vi "Aquire AI Data.vi"() -> ()   [LabVIEW 2017]
panel:
  out "Table":string[](array[string])
  out "Chart":dbl(graph)
  # "采集时间"
  # "采集棒位二进制值"
  # "查表输出值"
  # "棒位理论值"
  # "光栅尺位置"
  # "光栅尺速度"
  # "移动方向"
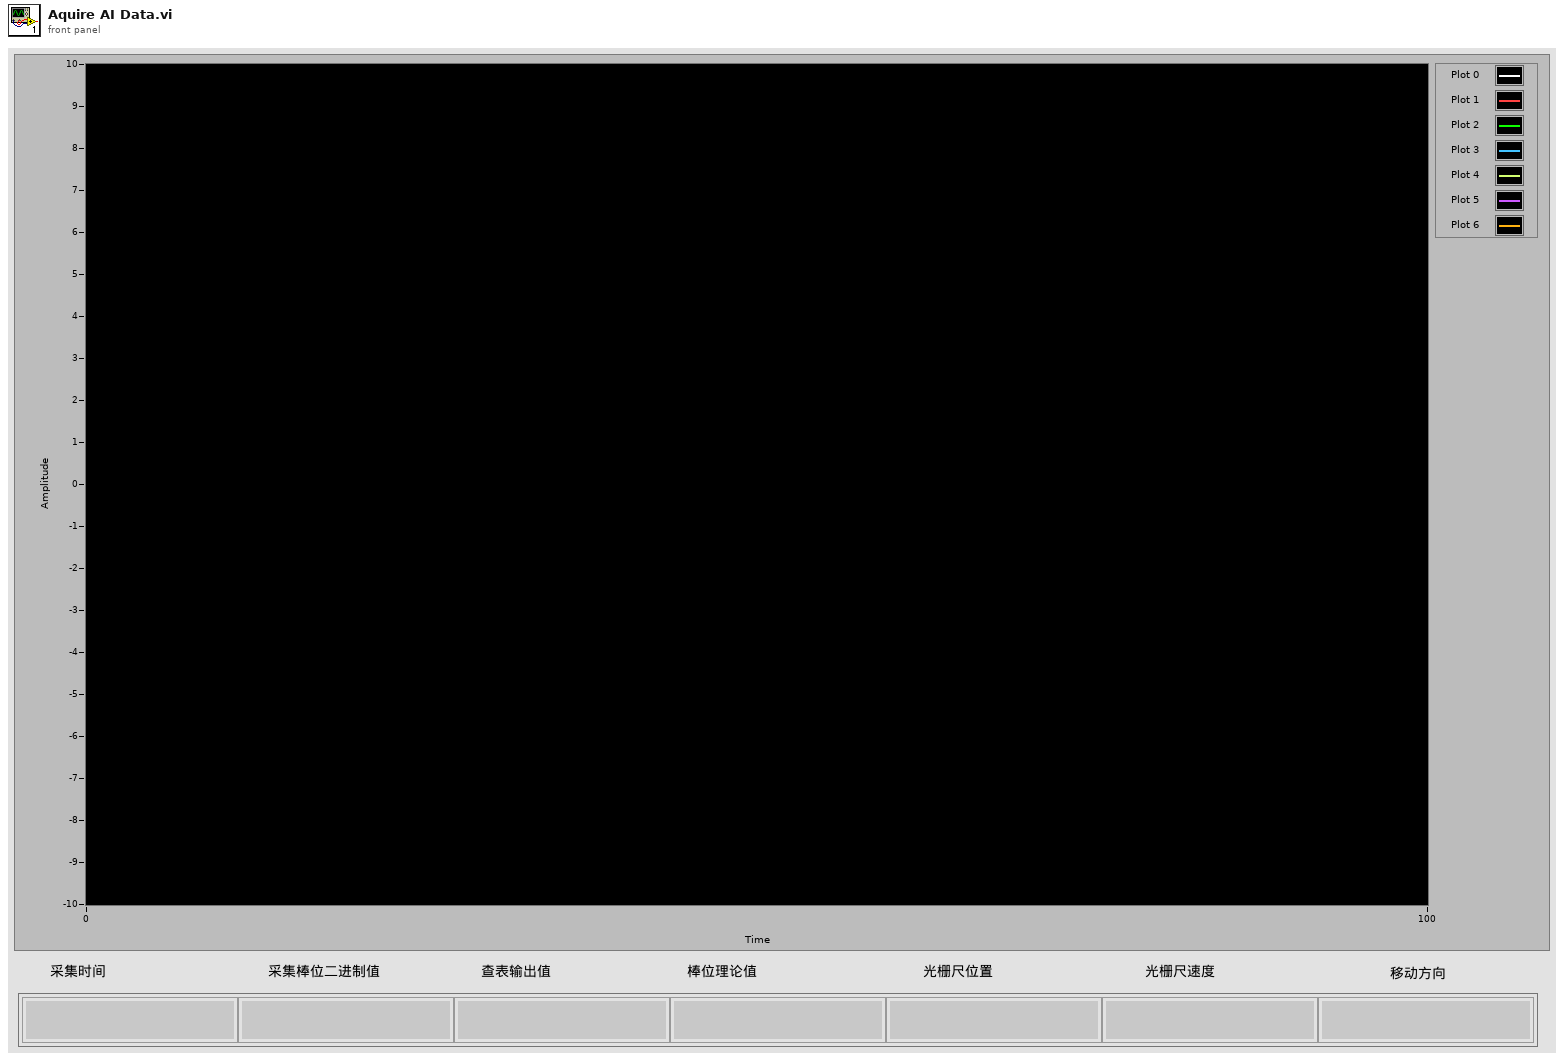
[diagram p1: front panel]
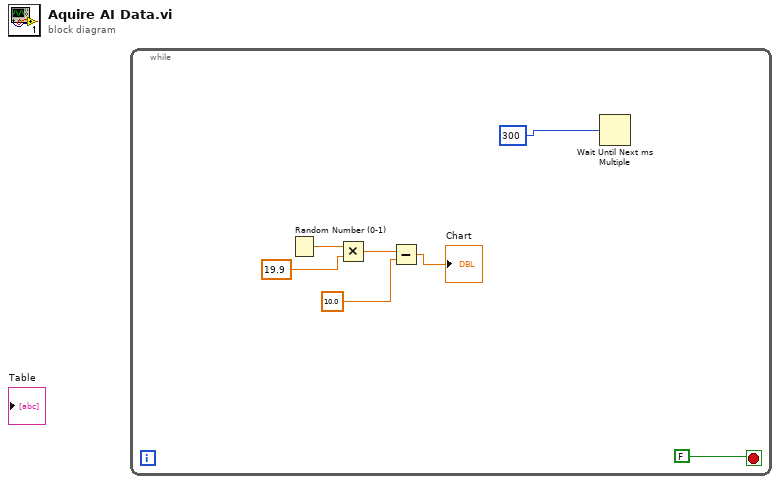
[diagram p0: block diagram]
diagram:
  n1 = while {
    stop <- FALSE stop-if-true
    n2 = Random Number (0-1)() -> (number: 0 to 1=w5:dbl)
    n3 = Multiply(x=w5, y=19.9) -> (x*y=w2:dbl)
    n4 = Subtract(x=w2, y=10.0) -> (x-y=→"Chart":dbl)
    n5 = Wait Until Next ms Multiple(millisecond multiple=300) -> ()  [unwired: 1 out]
  }
